vi "TestMatlabEvents.vi"() -> ()   [LabVIEW 2017]
panel:
  in  "Event Wait timeout":i32=10
  out "erros?":bool
  out "ExpID":string="Exp77c27ca2690b43b31b68791e85e1b449C"
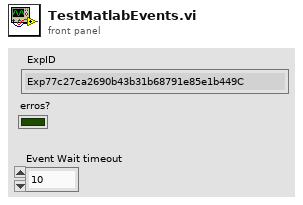
[diagram p1: front panel]
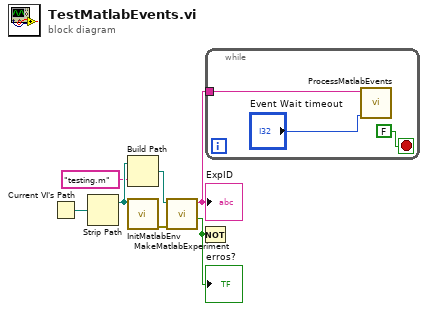
[diagram p0: block diagram]
diagram:
  n1 = Current VI's Path() -> (path=w4:path)
  n2 = Strip Path(path=w4) -> (stripped path=w6:path)  [unwired: 1 out]
  n3 = Build Path(base path=w6, name or relative path="testing.m") -> (appended path=w7:path)
  n4 = call "InitMatlabEnv.vi"("Working directory"=w6) -> ("error out"=w5:errorcluster)  [unwired: 10 in]
  n5 = call "MakeMatlabExperiment.vi"("error in"=w5, "experimentFilepath"=w7) -> ("erros?"=w2:bool, "ExpID"=w1:string)  [unwired: 6 in, 2 out]
  "ExpID" <- w1
  "erros?" <- w2
  n6 = Not(x=w2) -> ()  [unwired: 1 out]
  n7 = while {
    tunnel: w1 -> [w9]
    stop <- FALSE stop-if-true
    n8 = call "ProcessMatlabEvents.vi"("Event Wait timeout"="Event Wait timeout", "ExperimentID"=w9) -> ()  [unwired: 10 in]
  }
